vi "Parse PBC Telemetry.vi"(10 "Variant":variant) -> (2 "PBC Telemetry":T1 {"Raw_Telemetry" format="%04x"; "Register 0"."PBC_Rev" format="%02x"; "Register 0"."PBC_Fuse" format="%02x"; "Register 0"."PBC_ID" format="%02x"; "Register 1"."VSA_CPT" format="%02x"; "Register 2"."Saltaper" format="%01x"; "Register 3"."WDOG_Count" format="%04x"; "Register 3"."CRD_BDDR" format="%02x"; "Register 6"."CMD_A_VALID_CMD_CNT" format="%02x"; "Register 6"."CMD_A_INVALID" format="%02x"; "Register 7"."CMD_B_VALID_CMD_CNT" format="%02x"; "Register 7"."CMD_B_INVALID" format="%02x"; "Register 8"."Ki" format="%04x"; "Register 9"."Kp" format="%04x"; "Register 10"."Kd" format="%04x"; "Register 11"."VoltTapSp" format="%02x"; "Register 11"."CurrSp" format="%02x"; "Register 11"."voltSp" format="%02x"; "Register 12"."Reserved" format="%02x"; "Register 12"."IV_DAC" format="%04x"; "Register 15"."Vcps" format="%04x"; "Register 16"."AH_I_MSW" format="%04x"; "Register 17"."AH_I_LSW" format="%04x"; "Register 18"."Curr_Sp" format="%04x"; "Register 19"."DEBUG" format="%04x"})   [LabVIEW 2019]
panel:
  # "Volt Taper Setpoint"
  # "Current Setpoint"
  # "Volt Setpoint"
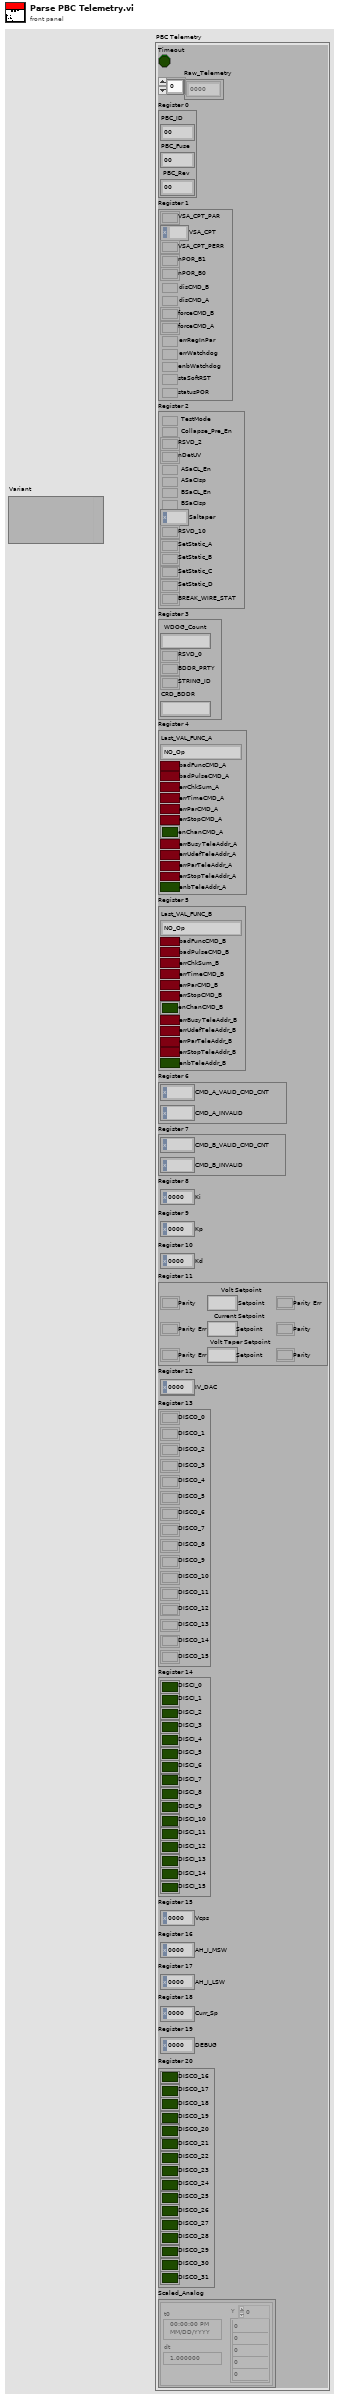
[diagram p1: front panel]
types:
  T1 = cluster{"Timeout":bool, "Raw_Telemetry":u16[], "Register 0":cluster{"PBC_ID":u8, "PBC_Fuse":u8, "PBC_Rev":u8}, "Register 1":cluster{"VSA_CPT_PAR":bool, "VSA_CPT":u8, "VSA_CPT_PERR":bool, "nPOR_B1":bool, "nPOR_B0":bool, "disCMD_B":bool, "disCMD_A":bool, "forceCMD_B":bool, "forceCMD_A":bool, "errRegInPar":bool, "errWatchdog":bool, "enbWatchdog":bool, "staSoftRST":bool, "statusPOR":bool}, "Register 2":cluster{"TestMode":bool, "Collapse_Pre_En":bool, "RSVD_2":bool, "nDetUV":bool, "ASaCL_En":bool, "ASaCIsp":bool, "BSaCL_En":bool, "BSaCIsp":bool, "Saltaper":u8, "RSVD_10":bool, "SetStatic_A":bool, "SetStatic_B":bool, "SetStatic_C":bool, "SetStatic_D":bool, "BREAK_WIRE_STAT":bool}, "Register 3":cluster{"CRD_BDDR":u8, "STRING_ID":bool, "BDDR_PRTY":bool, "RSVD_0":bool, "WDOG_Count":u16}, "Register 4":cluster{"Last_VAL_FUNC_A":enum16{"NO_Op", "Static_Discrete", "Housekeeping", "Memory_Command", "Bad_Command", "DynamicSwitch"}, "badFuncCMD_A":bool, "badPulseCMD_A":bool, "errChkSum_A":bool, "errTimeCMD_A":bool, "errParCMD_A":bool, "errStopCMD_A":bool, "enChanCMD_A":bool, "errBusyTeleAddr_A":bool, "errUdefTeleAddr_A":bool, "errParTeleAddr_A":bool, "errStopTeleAddr_A":bool, "enbTeleAddr_A":bool}, "Register 5":cluster{"Last_VAL_FUNC_B":enum16{"NO_Op", "Static_Discrete", "Housekeeping", "Memory_Command", "Bad_Command", "DynamicSwitch"}, "badFuncCMD_B":bool, "badPulseCMD_B":bool, "errChkSum_B":bool, "errTimeCMD_B":bool, "errParCMD_B":bool, "errStopCMD_B":bool, "enChanCMD_B":bool, "errBusyTeleAddr_B":bool, "errUdefTeleAddr_B":bool, "errParTeleAddr_B":bool, "errStopTeleAddr_B":bool, "enbTeleAddr_B":bool}, "Register 6":cluster{"CMD_A_INVALID":u8, "CMD_A_VALID_CMD_CNT":u8}, "Register 7":cluster{"CMD_B_INVALID":u8, "CMD_B_VALID_CMD_CNT":u8}, "Register 8":cluster{"Ki":u16}, "Register 9":cluster{"Kp":u16}, "Register 10":cluster{"Kd":u16}, "Register 11":cluster{"voltSpPar":bool, "voltSp":u8, "voltSpParErr":bool, "CurrSpPar":bool, "CurrSp":u8, "CurrSpParErr":bool, "VoltTapPar":bool, "VoltTapSp":u8, "VoltTapSpParErr":bool}, "Register 12":cluster{"IV_DAC":u16, "Reserved":u8}, "Register 13":cluster{"DISCO_0":bool, "DISCO_1":bool, "DISCO_2":bool, "DISCO_3":bool, "DISCO_4":bool, "DISCO_5":bool, "DISCO_6":bool, "DISCO_7":bool, "DISCO_8":bool, "DISCO_9":bool, "DISCO_10":bool, "DISCO_11":bool, "DISCO_12":bool, "DISCO_13":bool, "DISCO_14":bool, "DISCO_15":bool}, "Register 14":cluster{"DISCI_0":bool, "DISCI_1":bool, "DISCI_2":bool, "DISCI_3":bool, "DISCI_4":bool, "DISCI_5":bool, "DISCI_6":bool, "DISCI_7":bool, "DISCI_8":bool, "DISCI_9":bool, "DISCI_10":bool, "DISCI_11":bool, "DISCI_12":bool, "DISCI_13":bool, "DISCI_14":bool, "DISCI_15":bool}, "Register 15":cluster{"Vcps":u16}, "Register 16":cluster{"AH_I_MSW":u16}, "Register 17":cluster{"AH_I_LSW":u16}, "Register 18":cluster{"Curr_Sp":u16}, "Register 19":cluster{"DEBUG":u16}, "Register 20":cluster{"DISCO_16":bool, "DISCO_17":bool, "DISCO_18":bool, "DISCO_19":bool, "DISCO_20":bool, "DISCO_21":bool, "DISCO_22":bool, "DISCO_23":bool, "DISCO_24":bool, "DISCO_25":bool, "DISCO_26":bool, "DISCO_27":bool, "DISCO_28":bool, "DISCO_29":bool, "DISCO_30":bool, "DISCO_31":bool}, "Scaled_Analog":waveform(dbl)[]}
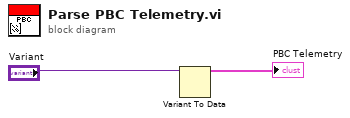
[diagram p0: block diagram]
diagram:
  n1 = Variant To Data(Variant="Variant") -> (data=→"PBC Telemetry":T1)  [unwired: 2 in, 1 out]
